vi "LWXPS_PositionerCorrectorP2IDFFAccelerationSet.vi"(0 "Integral gain 2":dbl, 1 "Derivative gain":dbl, 2 "Integral saturation value":dbl, 3 "Integration time":dbl, 4 "Derivative filter cut off frequency":dbl, 5 "Proportional gain multiplier":dbl, 6 "Integral gain multiplier":dbl, 7 "Derivative gain multiplier":dbl, 8 "Integral gain":dbl, 9 "Form coefficient":dbl, 10 "Proportional gain":dbl, 11 "Feed forward acceleration":dbl, 12 "Closed Loop Status":bool, 13 "Feed forward jerk":dbl, 14 "Positioner Name":string, 15 "Setpoint position delay":dbl, 16 "XPS Reference IN":refnum<k24>, 17 "LabVIEW error IN":errorcluster) -> (20 "XPS Reference OUT":refnum<k24>, 22 "Returned error code":i32, 25 "XPS Error String":string, 27 "LabVIEW error OUT":errorcluster)   [LabVIEW 2014]
uses:
  D:/XPSQ8_LabView_Library/Development/Source/Dll/Newport.XPS.CommandInterface.dll
  Dll/Newport.XPS.CommandInterface.dll
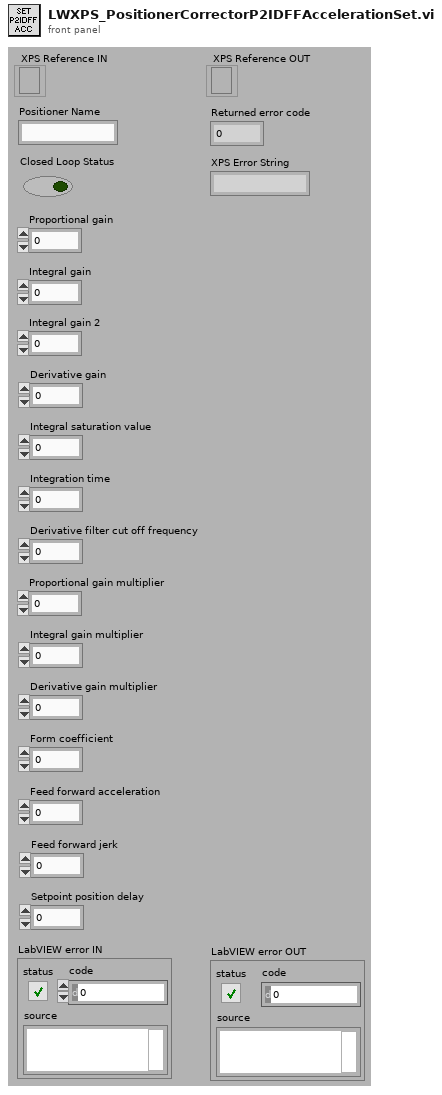
[diagram p1: front panel]
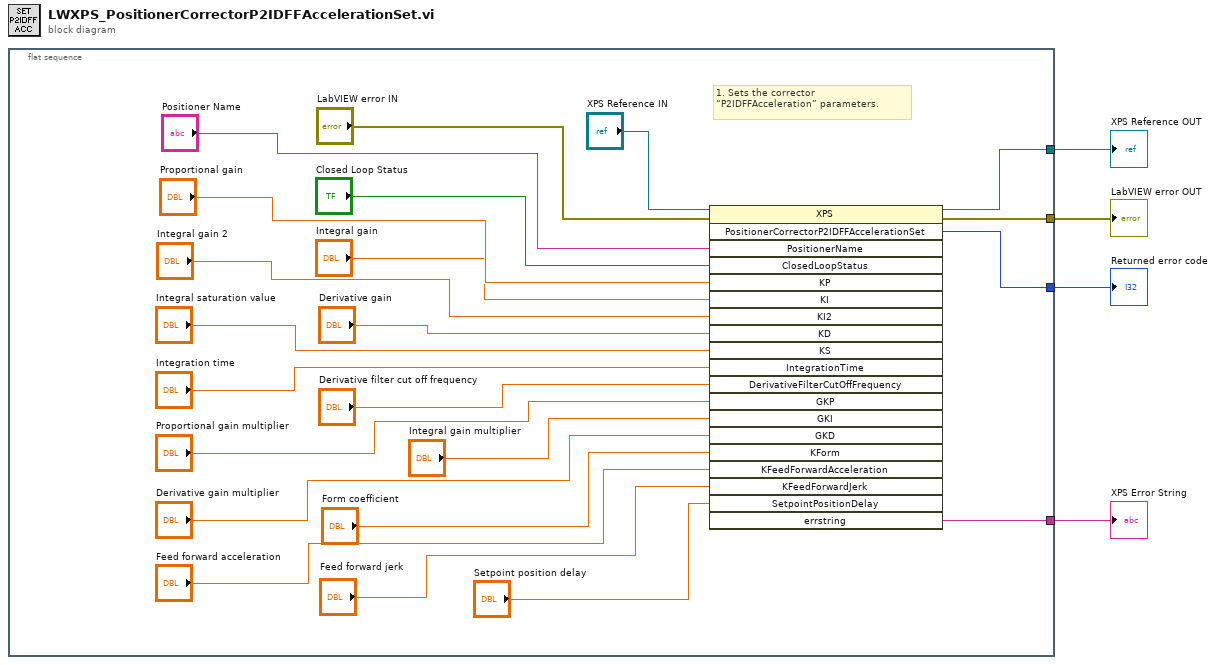
[diagram p0: block diagram]
diagram:
  n1 = flat-sequence {
    tunnel: [w22] -> w4
    tunnel: [w25] -> w3
    tunnel: [w24] -> w2
    tunnel: [w7] -> w1
    frame #0 {
      # "1. Sets the corrector “P2IDFFAcceleration” parameters."
      n2 = invoke class="XPS" method="PositionerCorrectorP2IDFFAccelerationSet"(reference="XPS Reference IN", error in="LabVIEW error IN", "PositionerName"="Positioner Name", "ClosedLoopStatus"="Closed Loop Status", "KP"="Proportional gain", "KI"="Integral gain", "KI2"="Integral gain 2", "KD"="Derivative gain", "KS"="Integral saturation value", "IntegrationTime"="Integration time", "DerivativeFilterCutOffFrequency"="Derivative filter cut off frequency", "GKP"="Proportional gain multiplier", "GKI"="Integral gain multiplier", "GKD"="Derivative gain multiplier", "KForm"="Form coefficient", "KFeedForwardAcceleration"="Feed forward acceleration", "KFeedForwardJerk"="Feed forward jerk", "SetpointPositionDelay"="Setpoint position delay") -> (reference out=w22:refnum<k24>, error out=w25:errorcluster, "PositionerCorrectorP2IDFFAccelerationSet"=w24:i32, "errstring"=w7:string)  [unwired: 2 in, 16 out]
    }
  }
  "XPS Error String" <- w1
  "XPS Reference OUT" <- w4
  "LabVIEW error OUT" <- w3
  "Returned error code" <- w2
